vi "Test 7 Get Game Number.vi"(8 "error in (no error)":errorcluster, 11 "Test Case In":refnum<class "Game Test.lvclass">) -> (0 "error out":errorcluster, 3 "Test Case Out":refnum<class "Game Test.lvclass">)   [LabVIEW 2020, in "Game Test.lvclass"]
uses:
  Game Test.lvclass
  C:/Program Files (x86)/National Instruments/LabVIEW 2020/vi.lib/Astemes/LUnit/Test Case.lvclass
  <vilib>/Astemes/LUnit/Test Case.lvclass/Test Case.ctl
  902a8a3b-ea14-456a-be5f-ae822212fefc.vi
  <vilib>/Astemes/LUnit/Append Pass Result.vi
  <vilib>/Astemes/LUnit/Append Fail Result.vi
  <vilib>/Astemes/LUnit/Describe Comparison.vi
  <vilib>/Astemes/LUnit/Compare Variants.vi
  <vilib>/Astemes/LUnit/Variant to string.vi
  <vilib>/Utility/Data Type/Get Type Information.vi
  <vilib>/Utility/LVClass/Get LV Class Name.vi
  Game/Game.lvclass
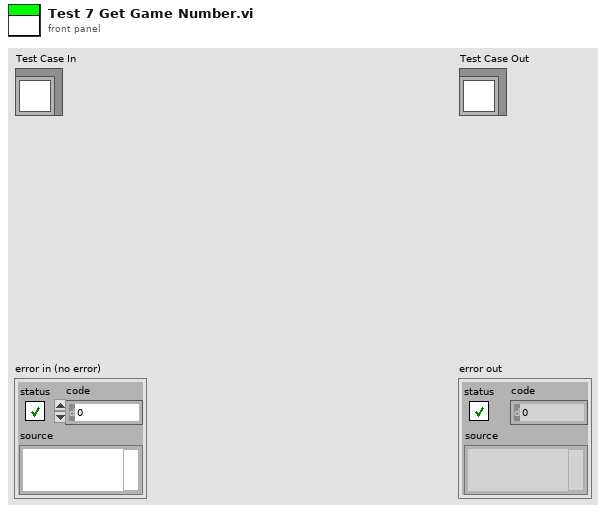
[diagram p1: front panel]
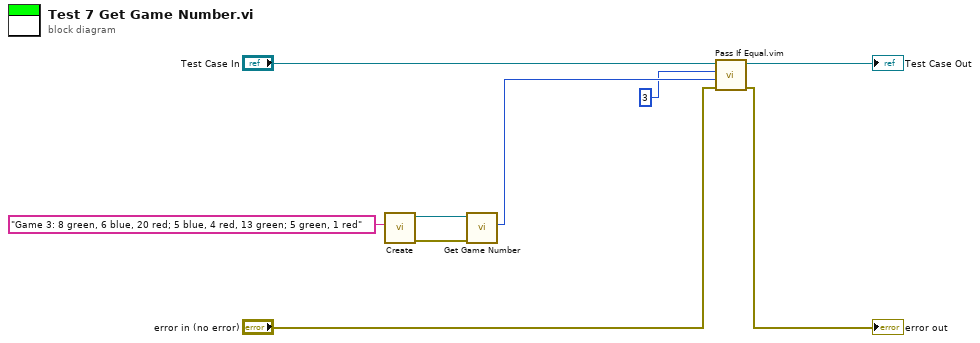
[diagram p0: block diagram]
diagram:
  n1 = call "Create.vi"("Input"="Game 3: 8 green, 6 blue, 20 red; 5 blue, 4 red, 13 green; 5 green, 1 red") -> ("error out"=w3:errorcluster, "Game"=w4:refnum<class "Game.lvclass">)  [unwired: 9 in]
  n2 = call "Get Game Number.vi"("error in (no error)"=w3, "Game in"=w4) -> ("Number"=w2:i32)  [unwired: 7 in, 2 out]
  n3 = call "Pass If Equal.vim"("error in (no error)"="error in (no error)", "Actual"=w2, "Expected"=3 ("Number"), "LUnit Test Case In"="Test Case In") -> ("error out"=→"error out":errorcluster, "LUnit Test Case Out"=→"Test Case Out":refnum<class "Game Test.lvclass">)  [unwired: 6 in]
